vi "HSE Application not initialized--error.vi"() -> (0 "error out":errorcluster)   [LabVIEW 2020, in "hse-application.lvclass"]
doc: "HSE Application not initialized\n\n____\nHAMPEL SOFTWARE ENGINEERING v3.8.0 (2023-12-18 14:41)"
uses:
  hse-application.lvclass
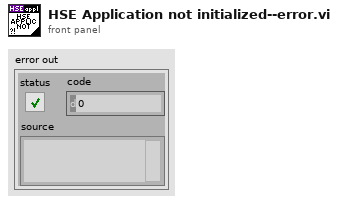
[diagram p1: front panel]
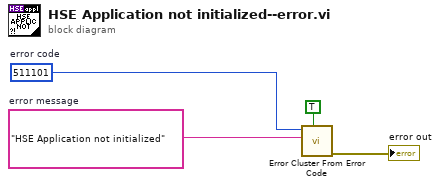
[diagram p0: block diagram]
diagram:
  w2 = "HSE Application not initialized"  # error message
  w3 = 511101  # error code
  n1 = call <vilib>:"Error Cluster From Error Code.vi"("show call chain? (False)"=TRUE, "error message (\"\")"=w2, "error code (0)"=w3) -> ("error out"=→"error out":errorcluster)  [unwired: 6 in]
